vi "CRYFlatten Scope-FFT.vi"(11 "Scope-FFT settings":T1={"window"=1, "n avgs"=1, "lin/exp avg"=0, "pwr/cplx avg"=0, "time (ms)"=0.05, "fft lines"=2048, "scope/fft mode"=0, "channel"=0, "trig. channel"=0, "Applay Correction"=FALSE, "Time Display"="%#_6p", "Freq. Weighting"="None", "Ave/Max/Min"=0, "Trigger Level"=0.0, "Trigger Unit"=0, "Trigger Time Offset"=0.0, "Trigger Slope"=0, "Trigger/Free Run"=TRUE, "continuous"=FALSE, "Spectrum Display"="%#_6p", "Calc FFT"=TRUE, "Y-axis"="dB", "Signal Type"=""} {"Trigger Time Offset" format="%.2f"; "Trigger Level" format="%.2f"; "time (ms)" format="%.2f"}) -> (3 "Flat Scope-FFT settings":string="%#_6p")   [LabVIEW 2013]
uses:
  Typedef Control/CRYScope-FFT.ctl
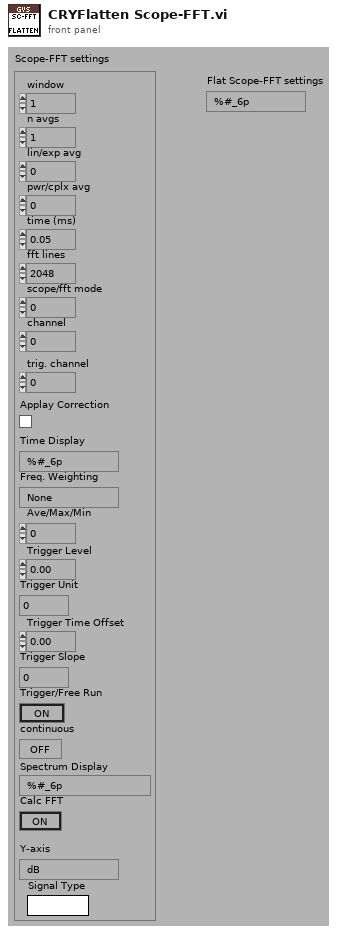
[diagram p1: front panel]
types:
  T1 = typedef "CRYScope-FFT.ctl" = cluster{"window":i32, "n avgs":i32, "lin/exp avg":i32, "pwr/cplx avg":i32, "time (ms)":dbl, "fft lines":i32, "scope/fft mode":i32, "channel":i32, "trig. channel":i32, "Applay Correction":bool, "Time Display":string, "Freq. Weighting":string, "Ave/Max/Min":u16, "Trigger Level":dbl, "Trigger Unit":u16, "Trigger Time Offset":dbl, "Trigger Slope":u16, "Trigger/Free Run":bool, "continuous":bool, "Spectrum Display":string, "Calc FFT":bool, "Y-axis":string, "Signal Type":string}
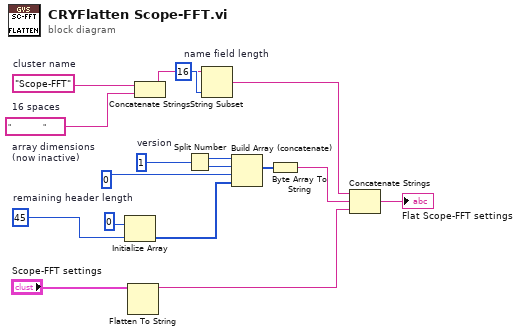
[diagram p0: block diagram]
diagram:
  w4 = u8 0  # array dimensions (now inactive)
  w7 = 16  # name field length
  w8 = "                "  # 16 spaces
  w9 = "Scope-FFT"  # cluster name
  w13 = 45  # remaining header length
  w17 = u16 1  # version
  n1 = Initialize Array(u8 0, w13) -> (w10:u8[])
  n2 = Flatten To String(anything="Scope-FFT settings") -> (data string=w3:string)  [unwired: 1 in, 4 out]
  n3 = Concatenate Strings(w9, w8) -> (w6:string)
  n4 = Split Number(x=w17) -> (hi(x)=w16:u8, lo(x)=w15:u8)
  n5 = String Subset(string=w6, length (rest)=w7) -> (substring=w5:string)  [unwired: 1 out]
  n6 = Build Array (concatenate)(w16, w15, w4, w10) -> (w12:u8[])
  n7 = Byte Array To String(unsigned byte array=w12) -> (string=w11:string)
  n8 = Concatenate Strings(w5, w11, w3) -> (→"Flat Scope-FFT settings":string)
